vi "rearrange.vi"(9 "units":string(combo), 10 "Points to Aquire":i32, 11 "Array in":dbl[][](array[numeric])) -> (0 "units":string[](array[string]), 1 "varnames":string[](array[string]), 3 "Array out":dbl[][](array[numeric]))   [LabVIEW 2017]
panel:
  out "String Array From File":string[][](array[string])
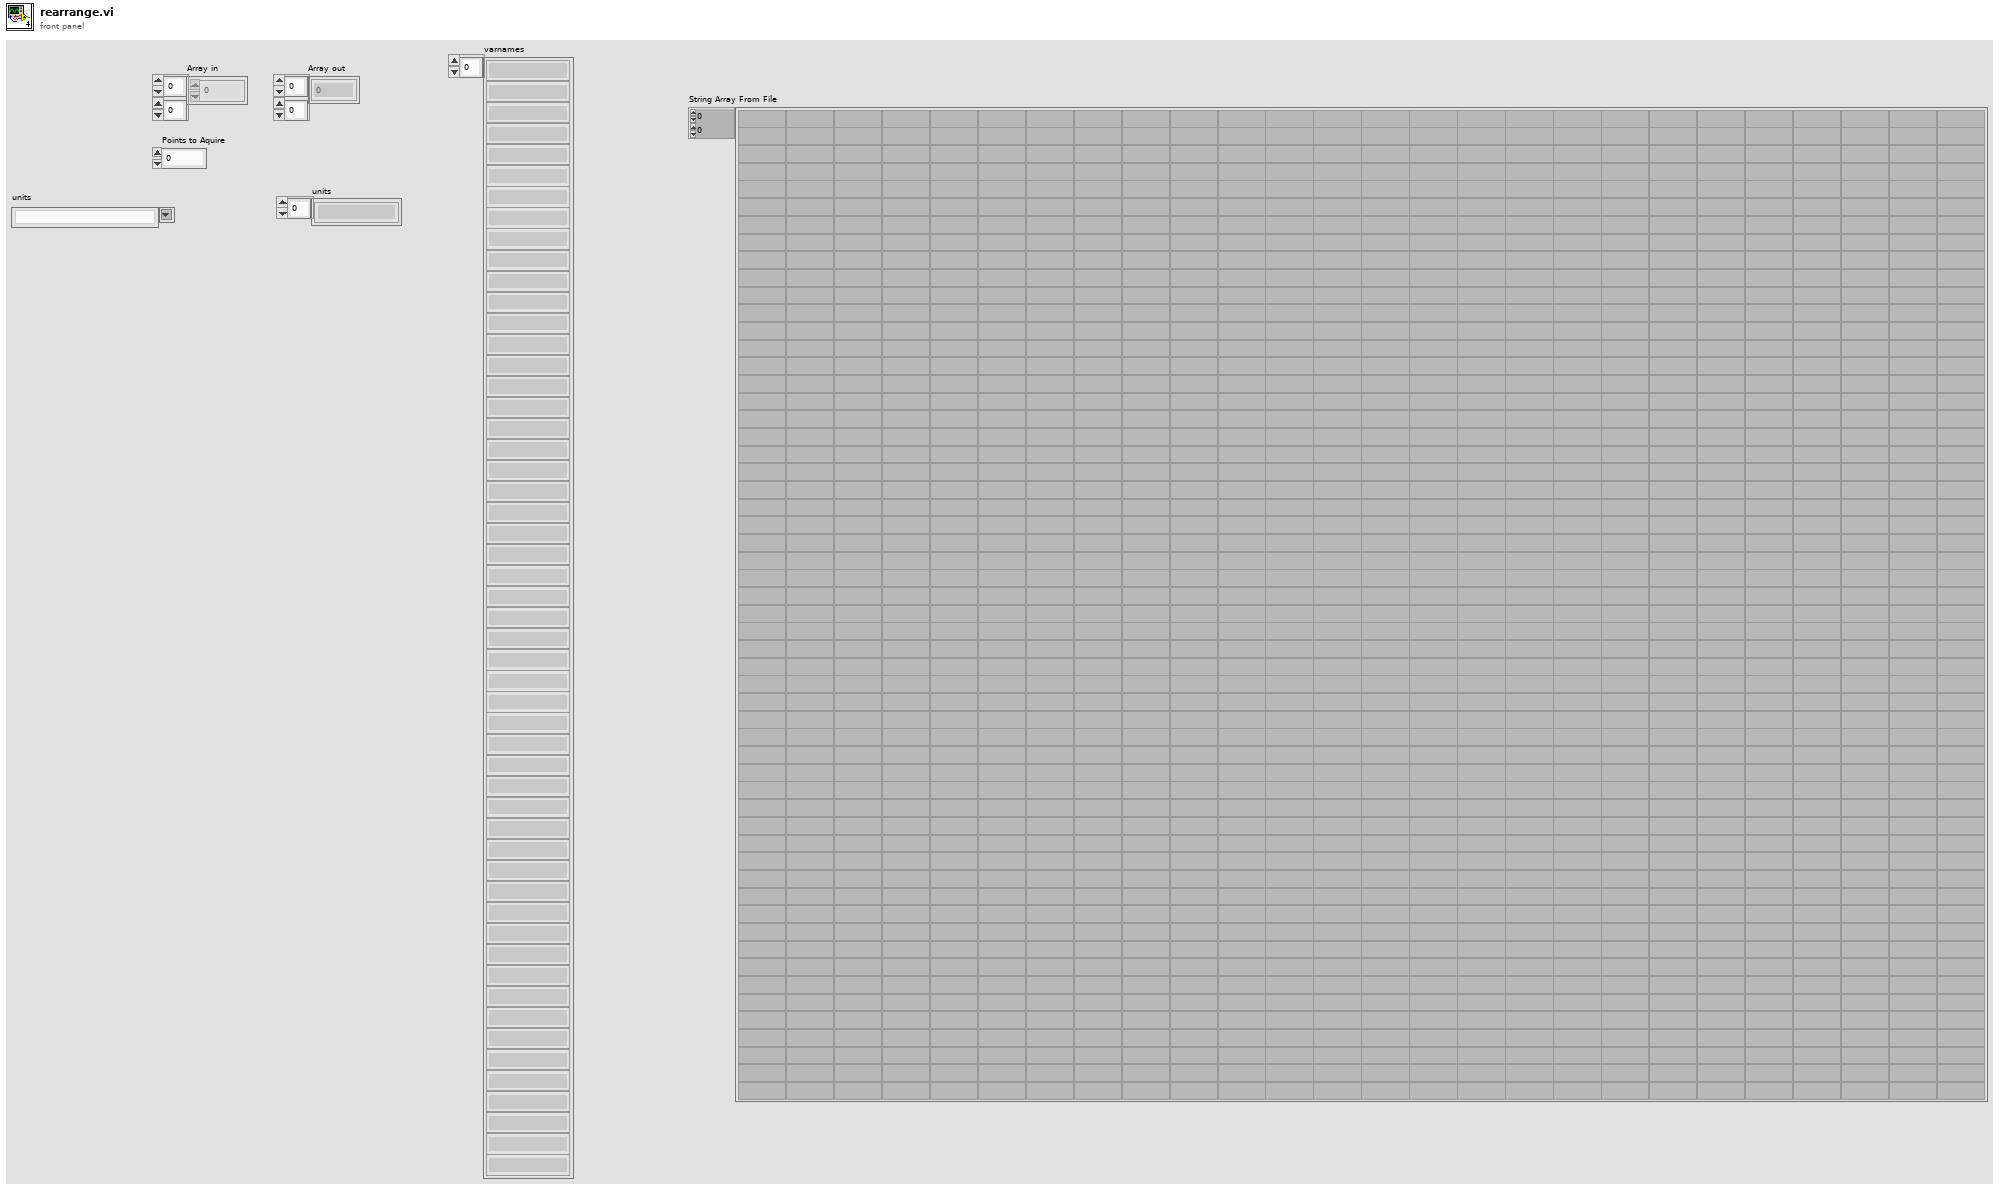
[diagram p1: front panel]
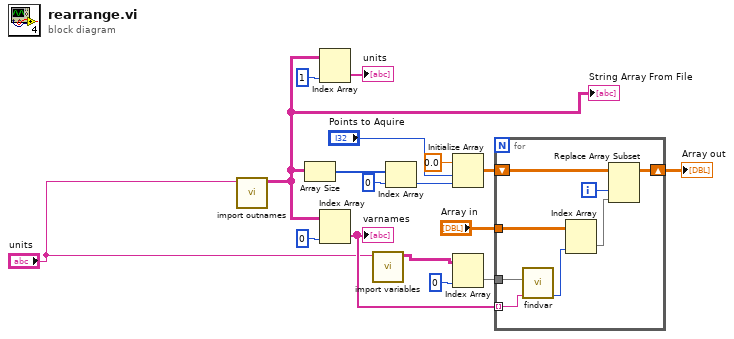
[diagram p0: block diagram]
diagram:
  n1 = call "import outnames.vi"("units"="units") -> ("String Array From File"=w3:string[][])  [unwired: 10 in]
  "String Array From File" <- w3
  n2 = Array Size(array=w3) -> (size(s)=w10:i32[])
  n3 = Index Array(array=w3, index (col)=1 ("disabled index (col)")) -> (element=→"units":string[])  [unwired: 1 in]
  n4 = Index Array(array=w3, index (col)=0 ("disabled index (col)")) -> (element=w6:string[])  [unwired: 1 in]
  "varnames" <- w6
  n5 = call "import variables.vi"("units"="units") -> ("String Array From File"=w2:string[][])  [unwired: 9 in, 1 out]
  n6 = Index Array(array=w10, index=0) -> (element=w13:i32)
  n7 = Initialize Array(0.0 ("element"), "Points to Aquire", w13) -> (w11:dbl[][])
  n8 = Index Array(array=w2, index (col)=0 ("disabled index (col)")) -> (element=w7:string[])  [unwired: 1 in]
  n9 = for {
    tunnel: w6 -> [w25] mode=indexing
    tunnel: w7 -> [w24]
    tunnel: "Array in" -> [w20]
    shift-right: [w21] -> w15
    shift-left: w11 -> [w23]
    i -> [w22]
    n10 = call "findvar.vi"("varin"=w25, "varnames"=w24) -> ("indexno"=w19:i32)  [unwired: 8 in, 1 out]
    n11 = Index Array(array=w20, index (col)=w19) -> (element=w18:dbl[])  [unwired: 1 in]
    n12 = Replace Array Subset(array=w23, new element=w18, index (col)=w22) -> (w21:dbl[][])  [unwired: 1 in]
  }
  "Array out" <- w15
